vi "chkItemFoundInTree.vi"(8 "error in":errorcluster, 10 "searchItem":string, 11 "Tree Refnum in":refnum<vi>) -> (0 "error out":errorcluster, 2 "FoundInTree?":bool, 3 "Tree Refnum out":refnum<vi>)   [LabVIEW 2010]
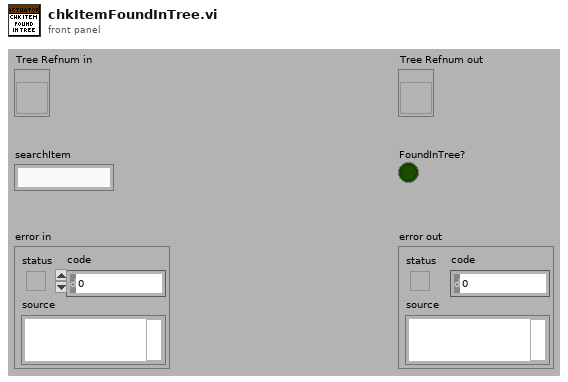
[diagram p1: front panel]
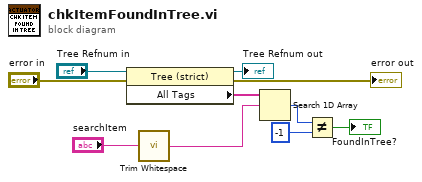
[diagram p0: block diagram]
diagram:
  n1 = property on="Property Node" class="Tree (strict)"(reference="Tree Refnum in", error in="error in") -> (reference out=→"Tree Refnum out":refnum<vi>, error out=→"error out":errorcluster, "All Tags"=w9:string[])
  n2 = call <vilib>:"Trim Whitespace.vi"("string"="searchItem") -> ("trimmed string"=w1:string)  [unwired: 1 in]
  n3 = Search 1D Array(1D array=w9, element=w1) -> (index of element=w7:i32)  [unwired: 1 in]
  n4 = Not Equal?(x=w7, y=-1) -> (x != y?=→"FoundInTree?":bool)
